vi "Read Single-Point Core.vi"(8 "error in (no error)":errorcluster, 10 "maximum time (5s)":dbl[unit]=5.0 caption="maximum time (5000 ms)", 11 "IVI_DMM_Delayed in":refnum<class "IVI_DMM_Delayed.lvclass">) -> (0 "error out":errorcluster, 2 "reading":dbl format="%^.2e", 3 "IVI_DMM_Delayed out":refnum<class "IVI_DMM_Delayed.lvclass">)   [LabVIEW 2015, in "IVI_DMM.lvlib" / "IVI_DMM_Delayed.lvclass"]
doc: "This VI initiates a measurement, waits until the DMM has returned to the Idle state, and returns the measured value.\n\nThis VI applies default values to properties that have not been set by the user under the following conditions:\n\n(1) If the user has not set the value of any property in the IviDmmMultiPoint extension group, the VI sets the IviDmm>>Multi-Point Acquisition>>Sample Count [MP] and IviDmm>>Multi-Point Acquisition>>Trigger Count [MP] properties to 1.\n\n(2) If the user has not set the value of the IviDmm>Measurement Operation Options>Auto Zero [AZ] property, the VI sets the value of this property to IVIDMM_VAL_AUTO_ZERO_OFF (0). \n\nNotes:\n\n(1) After this VI executes, the Reading parameter contains an actual reading or a value indicating that an over-range condition occurred.\n\n(2) If an over-range condition occurs, the Reading parameter contains an IEEE defined NaN (Not a Number) value and the VI returns the IVIDMM_WARN_OVER_RANGE (0x3ffA2001) warning code.\n\n(3) You can test the measurement value for an over-range condition by calling the IviDmm Is Over-Range VI.\n\n(4) This VI performs interchangeability checking when the IviDmm>>Inherent IVI Settings>>User Options>>Interchange Check property is set to TRUE. If the IviDmm>>Inherent IVI Settings>>User Options>>Spy property is set to TRUE, you use the NI Spy utility to view interchangeability warnings. You use the IviDmm Get Next Interchange Warning VI to retrieve interchangeability warnings when the IviDmm>>Inherent IVI Settings>>User Options>>Spy property is set to FALSE. For more information about interchangeability checking, refer to the help text for the IviDmm>>Inherent IVI Settings>>User Options>>Interchange Check property.\n\n(5) The class driver returns a simulated measurement when this VI is called and the IviDmm>>Inherent IVI Settings>>User Options>>Simulate property is set to TRUE and the IviDmm>>Inherent IVI Settings>>User Options>>Use Specific Simulation property is set to FALSE. For information on how to configure a simulated measurement, refer to the online help manual."
uses:
  IVI_DMM_Delayed.lvclass
  IVI_DMM_Delayed.lvclass/IVI_DMM_Delayed.ctl
  IVI_DMM/IVI_DMM.lvclass
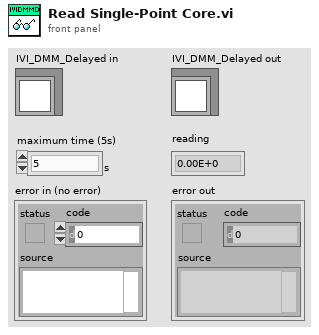
[diagram p1: front panel]
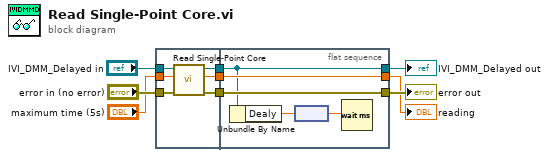
[diagram p0: block diagram]
diagram:
  n1 = flat-sequence {
    tunnel: "error in (no error)" -> [w12]
    tunnel: "maximum time (5s)" -> [w11]
    tunnel: "IVI_DMM_Delayed in" -> [w10]
    tunnel: [w15] -> w3
    tunnel: [w14] -> w2
    tunnel: [w13] -> w1
    tunnel: [w16] -> w7
    tunnel: [w19] -> w8
    tunnel: [w20] -> w9
    tunnel: w3 -> [w20]
    tunnel: w2 -> [w19]
    tunnel: w1 -> [w16]
    frame #0 {
      n2 = call-parent "Read Single-Point Core.vi"("error in (no error)"=w12, "maximum time (5s)"=w11, "IVI_DMM in"=w10) -> ("error out"=w15:errorcluster, "reading"=w14:dbl, "IVI_DMM out"=w13:refnum<class "IVI_DMM_Delayed.lvclass">)  [unwired: 6 in]
    }
    frame #1 {
      n3 = Unbundle By Name(w16) -> ("Dealy"=w17:dbl[unit])
      n4 = node(w17) -> (w18:dbl)
      n5 = Wait (ms)(milliseconds to wait=w18) -> ()  [unwired: 1 out]
    }
  }
  "error out" <- w9
  "IVI_DMM_Delayed out" <- w7
  "reading" <- w8
